vi "Configure PRACH Repetition.vi"(8 "error in (no error)":errorcluster, 9 "Repetition (Single shot measurement)":i32(ring) items=["Single shot measurement", "Continuous measurement"], 10 "Instance (1)":T1=1, 11 "VISA resource name":refnum<visa-resource-name>) -> (0 "error out":errorcluster, 3 "VISA resource name out":refnum<visa-resource-name>)   [LabVIEW 2020, in "Rohde&Schwarz CMWXP NR FR1 Measurement.lvlib"]
doc: "Specifies the repetition mode of the measurement. The repetition mode specifies whether the measurement is stopped after a single shot or repeated continuously. Use CONFigure:..:MEAS<i>:...:SCOunt to determine the number of measurement intervals per single shot.\n\nAttribute:\nRSCMWXPNRFR1M_ATTR_PRACH_REPETITION\n\nRemote-control command:\nCONFigure:NRSub:MEAS<i>:PRACh:REPetition"
uses:
  <instrlib>/Rohde&Schwarz CMWXP NR FR1 Measurement/Rohde&Schwarz CMWXP NR FR1 Measurement.lvlib
  <instrlib>/Rohde&Schwarz CMWXP NR FR1 Measurement/Private/_Instance.ctl
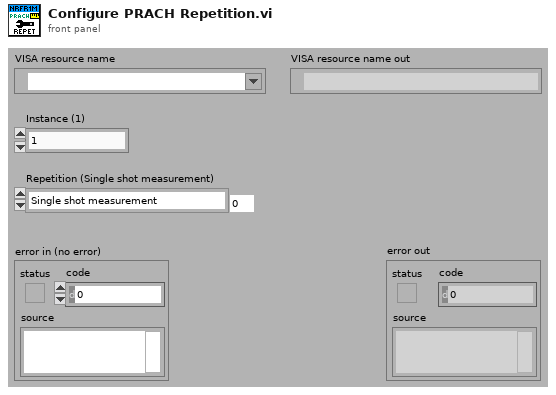
[diagram p1: front panel]
types:
  T1 = typedef "Rohde&Schwarz CMWXP NR FR1 Measurement.lvlib/_Instance.ctl" = i32
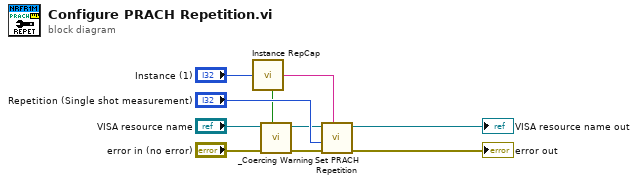
[diagram p0: block diagram]
diagram:
  n1 = call <instrlib>:"Instance RepCap.vi"("Instance In"="Instance (1)") -> ("In Range?"=w2:bool, "RepCap Identifier Out"=w1:string)  [unwired: 1 in]
  n2 = call <instrlib>:"_Coercing Warning.vi"("In Range?"=w2, "error in (no error)"="error in (no error)", "VISA resource name"="VISA resource name") -> ("error out"=w5:errorcluster, "VISA resource name out"=w4:refnum<visa-resource-name>)  [unwired: 7 in]
  n3 = call "Set PRACH Repetition"("Repeated Capabilities"=w1, "error in (no error)"=w5, "PRACH Repetition (0 - Single shot measurement)"="Repetition (Single shot measurement)", "instrument handle"=w4) -> ("error out"=→"error out":errorcluster, "instrument handle out"=→"VISA resource name out":refnum<visa-resource-name>)  [unwired: 6 in]
